vi "Simulation VI.vi"() -> ()   [LabVIEW 2015, in "Simulation.lvlib"]
uses:
  Simulation.lvlib
  Simulation Data_Global.vi
panel:
  in  "Fan B Fault":bool
  in  "Fan A Fault":bool
  in  "stop":bool
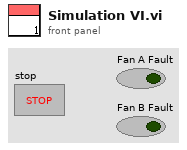
[diagram p1: front panel]
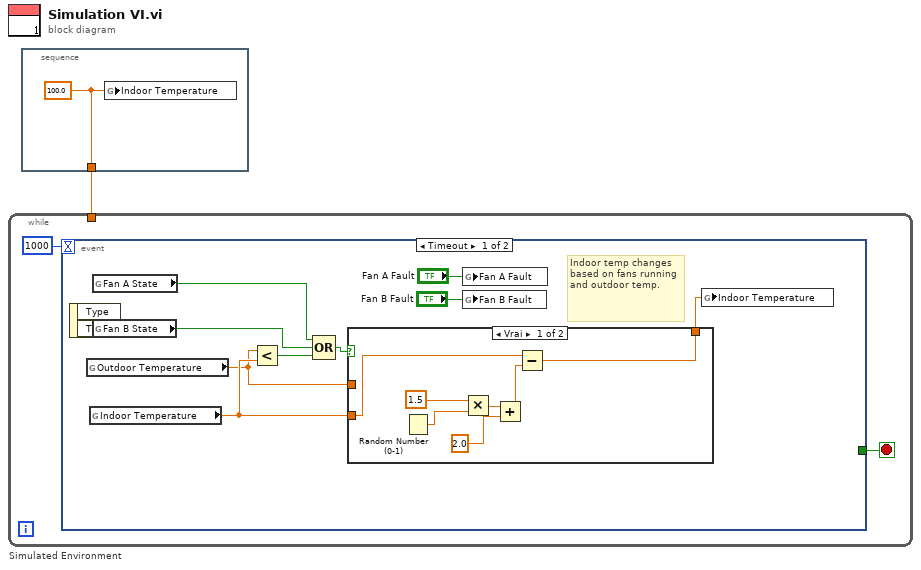
[diagram p0: block diagram]
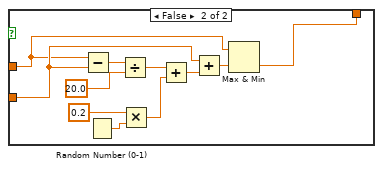
[diagram p2: hidden frame]
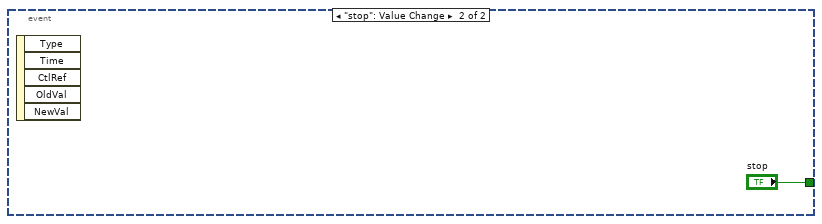
[diagram p3: hidden frame]
diagram:
  n1 = stacked-sequence {
    tunnel: [w2] -> w1
    frame #0 {
      w2 = 100.0 ("Temperature")
      n2 = global write "Simulation Data_Global.vi" "Indoor Temperature"(w2) -> ()
    }
  }
  n3 = while "Simulated Environment" {
    tunnel: w1 -> [_]
    stop <- w3 stop-if-true
    n4 = event shown="[0] Timeout" {
      selector: _ -> [_ _]
      dyn-events: _ -> [_ _]
      timeout: u32 1000 ("milliseconds to wait") -> [_ _]
      tunnel: [_ "stop"] -> w3
      event Timeout {
        # "Indoor temp changes based on fans running and outdoor temp."
        n5 = event-data() -> ()  [unwired: 1 in, 2 out]
        n6 = global read "Simulation Data_Global.vi" "Outdoor Temperature"() -> (w10:dbl)
        n7 = global read "Simulation Data_Global.vi" "Indoor Temperature"() -> (w11:dbl)
        n8 = global read "Simulation Data_Global.vi" "Fan A State"() -> (w9:bool)
        n9 = global read "Simulation Data_Global.vi" "Fan B State"() -> (w8:bool)
        n10 = Less?(x=w10, y=w11) -> (x < y?=w12:bool)
        n11 = Compound Arithmetic op=OR(w9, w8, w12) -> (w13:bool)
        n12 = case shown="Vrai" w13 {
          tunnel: w11 -> [w15 w23]
          tunnel: w10 -> [_ w22]
          tunnel: [w14 w21] -> w7
          frame True {
            n13 = Random Number (0-1)() -> (number: 0 to 1=w19:dbl)
            n14 = Multiply(x=1.5 ("y"), y=w19) -> (x*y=w18:dbl)
            n15 = Add(x=w18, y=2.0) -> (x+y=w16:dbl)
            n16 = Subtract(x=w15, y=w16) -> (x-y=w14:dbl)
          }
          frame False {
            n17 = Subtract(x=w22, y=w23) -> (x-y=w31:dbl)
            n18 = Random Number (0-1)() -> (number: 0 to 1=w27:dbl)
            n19 = Divide(x=w31, y=20.0) -> (x/y=w29:dbl)
            n20 = Multiply(x=0.2, y=w27) -> (x*y=w26:dbl)
            n21 = Add(x=w29, y=w26) -> (x+y=w25:dbl)
            n22 = Add(x=w23, y=w25) -> (x+y=w24:dbl)
            n23 = Max & Min(x=w22, y=w24) -> (min(x,y)=w21:dbl)  [unwired: 1 out]
          }
        }
        n24 = global write "Simulation Data_Global.vi" "Fan A Fault"("Fan A Fault") -> ()
        n25 = global write "Simulation Data_Global.vi" "Fan B Fault"("Fan B Fault") -> ()
        n26 = global write "Simulation Data_Global.vi" "Indoor Temperature"(w7) -> ()
      }
      event "stop": Value Change {
        n27 = event-data() -> ()  [unwired: 1 in, 5 out]
      }
    }
  }
